vi "Read Config URL.vi"(8 "error in (no error)":errorcluster, 11 "ViewableActor in":refnum<class "ViewableActor.lvclass">) -> (0 "error out":errorcluster, 2 "Config URL":string, 3 "ViewableActor out":refnum<class "ViewableActor.lvclass">)   [LabVIEW 2014, in "ViewableActor.lvlib" / "ViewableActor.lvclass"]
uses:
  ViewableActor.lvclass
  ViewableActor.lvclass/ViewableActor.ctl
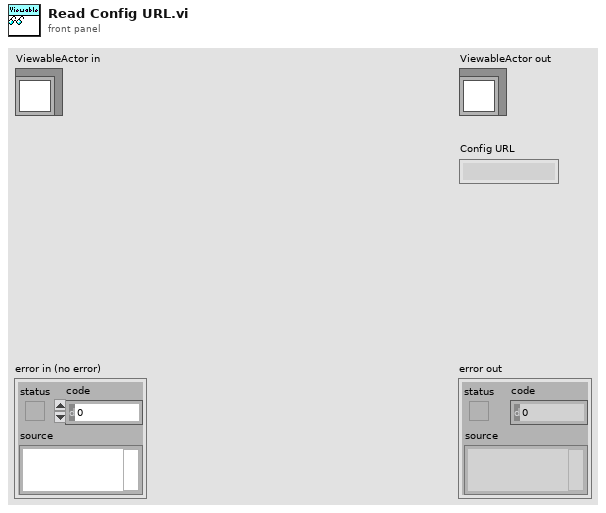
[diagram p1: front panel]
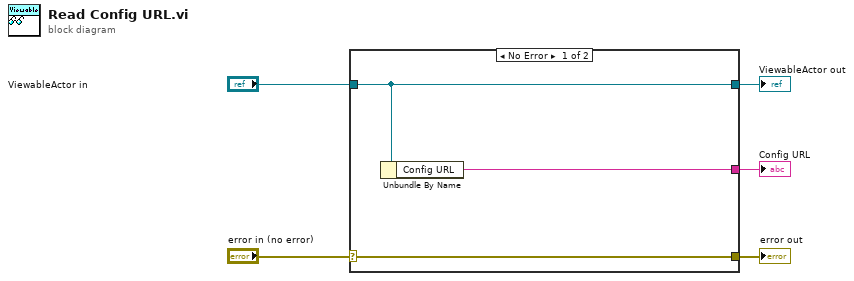
[diagram p0: block diagram]
diagram:
  n1 = case shown="No Error" "error in (no error)" {
    selector: "error in (no error)" -> [w8 w9]
    tunnel: [w8 w9] -> w4
    tunnel: [w7 w10] -> w2
    tunnel: "ViewableActor in" -> [w7 w10]
    tunnel: [w6 _] -> w1
    frame No Error {
      n2 = Unbundle By Name(w7) -> ("Config URL"=w6:string)
    }
    frame Error {
    }
  }
  "error out" <- w4
  "ViewableActor out" <- w2
  "Config URL" <- w1
